vi "Initialize Tag Tree.vi"(8 "error in (no error)":errorcluster, 10 "Tag Tree Helper":refnum<class "Tag Tree Helper.lvclass">, 11 "New Class Dialog In":refnum<class "New Class Dialog.lvclass">) -> (0 "error out":errorcluster, 3 "New Class Dialog Out":refnum<class "New Class Dialog.lvclass">)   [LabVIEW 2020, in "Process Generation.lvlib" / "New Class Dialog.lvclass"]
uses:
  New Class Dialog.lvclass
  Tag Tree Helper/Tag Tree Helper.lvclass
  New Class Dialog.lvclass/New Class Dialog.ctl
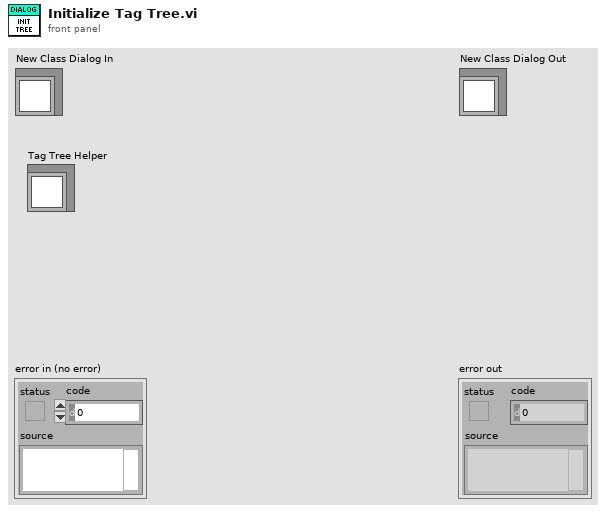
[diagram p1: front panel]
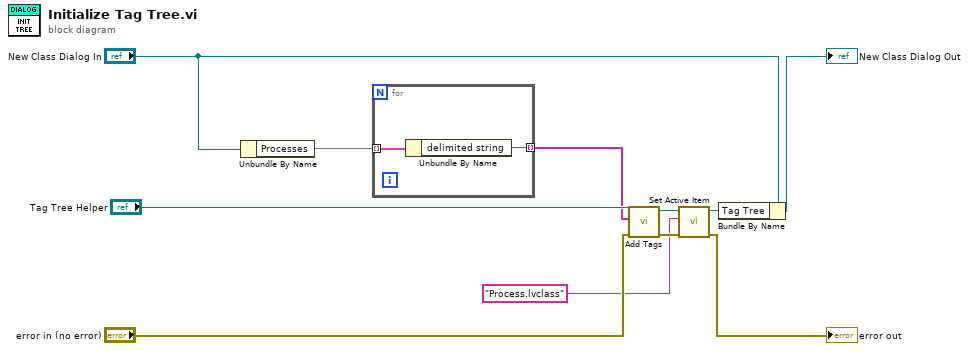
[diagram p0: block diagram]
diagram:
  n1 = Unbundle By Name("New Class Dialog In") -> ("Processes"=w10:map{string, path})
  n2 = for {
    tunnel: w10 -> [w13] mode=indexing
    tunnel: [w12] -> w8 mode=indexing
    n3 = Unbundle By Name(w13) -> ("delimited string"=w12:string)
  }
  n4 = call "Add Tags.vi"("error in (no error)"="error in (no error)", "Tag"=w8, "Tag Tree Helper In"="Tag Tree Helper") -> ("error out"=w3:errorcluster, "Tag Tree Helper Out"=w5:refnum<class "Tag Tree Helper.lvclass">)  [unwired: 7 in]
  n5 = call "Set Active Item.vi"("error in (no error)"=w3, "Tag"="Process.lvclass" ("Simple Name"), "Tag Tree Helper In"=w5) -> ("error out"=→"error out":errorcluster, "Tag Tree Helper Out"=w4:refnum<class "Tag Tree Helper.lvclass">)  [unwired: 7 in]
  n6 = Bundle By Name(cluster="New Class Dialog In", "Tag Tree"=w4) -> (→"New Class Dialog Out":refnum<class "New Class Dialog.lvclass">)
